vi "api_mqttDisconnect.vi"(0 "mqtt.lvclass in":refnum<class "mqtt.lvclass">, 11 "error in (no error)":errorcluster) -> (4 "mqtt.lvclass out":refnum<class "mqtt.lvclass">, 6 "success":bool, 15 "error out":errorcluster)   [LabVIEW 2018, in "labview-mqtt.lvlib" / "mqtt.lvclass"]
uses:
  mqtt.lvclass
  mqttTypedef/mqttQOSlevel.ctl
  mqttTypedef/mqttMessageType.ctl
  mqttCmd/mqttCmdDisconnect/mqttCmdDisconnect.lvclass
  D:/OneDrive/_WorkingOn/IECube/MQTT LabVIEW/mqtt-LabVIEW-master-yao/src/class/mqtt/mqttCmd/mqttCmd.lvclass
  mqttCmd/mqttCmd.lvclass/mqttCmd.ctl
  mqttCmd/mqttCmd.lvclass
  labview-mqtt.lvlib
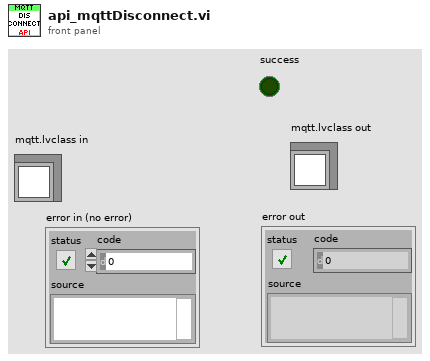
[diagram p1: front panel]
types:
  T1 = typedef "labview-mqtt.lvlib/mqttMessageType.ctl" = enum32{"Reserved", "CONNECT", "CONNACK", "PUBLISH", "PUBACK", "PUBREC", "PUBREL", "PUBCOMP", "SUBSCRIBE", "SUBACK", "UNSUBSCRIBE", "UNSUBACK", "PINGREQ", "PINGRESP", "DISCONNECT", "Reserved2"}
  T2 = typedef "labview-mqtt.lvlib/mqttQOSlevel.ctl" = enum8{"At most once", "At least once", "Exactly once", "Reserved"}
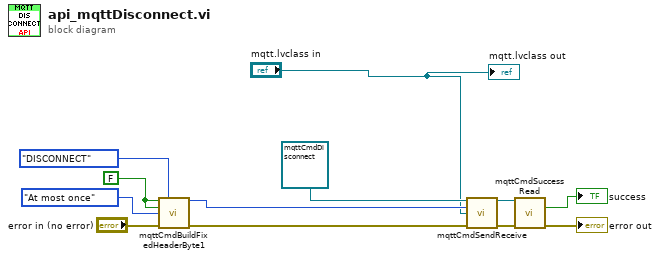
[diagram p0: block diagram]
diagram:
  w9 = FALSE
  n1 = call "mqttCmdBuildFixedHeaderByte1.vi"("retain(F)"=w9, "MessageType"=mqttMessageType."DISCONNECT", "duplicate(F)"=w9, "QoS (At most once)"=mqttQOSlevel."At most once", "error in (no error)"="error in (no error)") -> ("byte1"=w11:u8, "error out"=w7:errorcluster)  [unwired: 9 in]
  n2 = call "mqttCmdSendReceive.vi"("mqttConnect in"=refnum<class "mqttCmdDisconnect.lvclass"> refnum ("mqttBrokerCommandDisconnect.lvclass"), "byte1"=w11, "mqtt in"="mqtt.lvclass in", "error in (no error)"=w7) -> ("mqttConnect out"=w5:refnum<class "mqttCmdDisconnect.lvclass">, "error out"=w6:errorcluster)  [unwired: 9 in, 1 out]
  n3 = call "mqttCmdSuccessRead.vi"("mqttBrokerCommand in"=w5, "error in (no error)"=w6) -> ("success"=→"success":bool, "error out"=→"error out":errorcluster)  [unwired: 11 in, 1 out]
  "mqtt.lvclass out" <- "mqtt.lvclass in"
